vi "IR - Stop - addon.vi"(10 "IR Sensors":dbl[](array[numeric]), 11 "element":T1) -> (2 "appended array":dbl[](array[numeric]), 3 "0, 1":i16)   [LabVIEW 2019]
panel:
  out "Min":dbl
  out "Max":dbl
  out "logical AND":bool
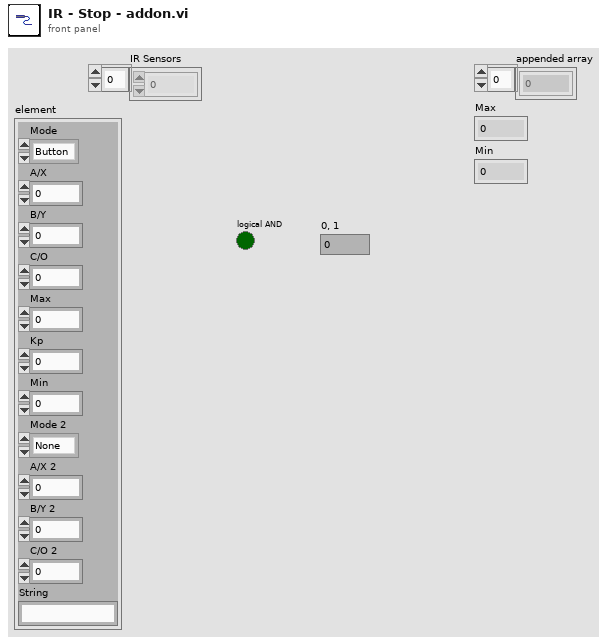
[diagram p1: front panel]
types:
  T1 = cluster{"Mode":enum16{"Button", "Encoder", "Delay", "IR Stop", "Line Stop"}, "A/X":dbl, "B/Y":dbl, "C/O":dbl, "Max":dbl, "Kp":dbl, "Min":dbl, "Mode 2":enum16{"None", "IR Stabilize", "Line Stabilize", "Encoder", "IR Stop", "Servo"}, "A/X 2":dbl, "B/Y 2":dbl, "C/O 2":dbl, "String":string}
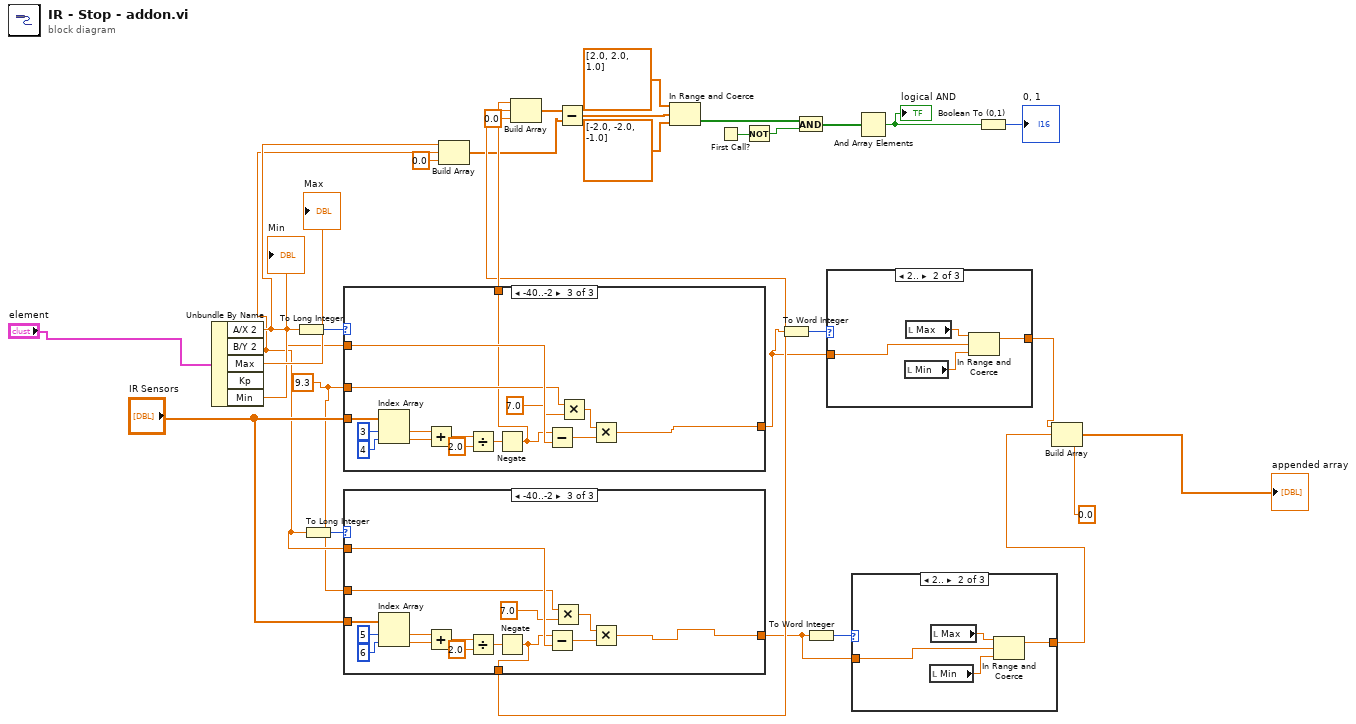
[diagram p0: block diagram]
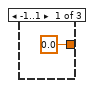
[diagram p2: hidden frame]
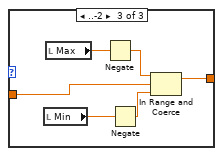
[diagram p3: hidden frame]
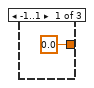
[diagram p4: hidden frame]
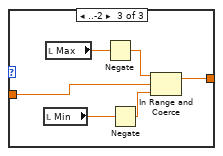
[diagram p5: hidden frame]
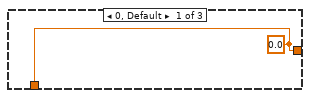
[diagram p6: hidden frame]
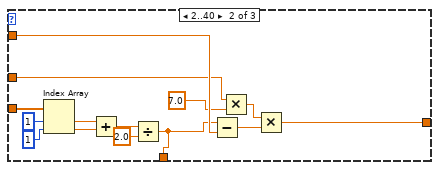
[diagram p7: hidden frame]
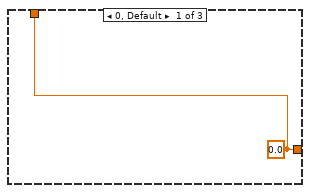
[diagram p8: hidden frame]
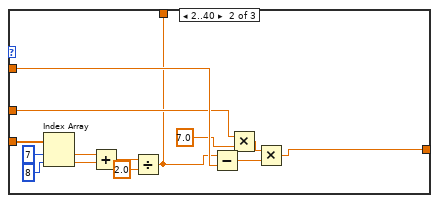
[diagram p9: hidden frame]
diagram:
  w2 = 9.3 ("Kp")
  n1 = Unbundle By Name("element") -> ("A/X 2"=w7:dbl, "B/Y 2"=w6:dbl, "Max"=→"Max":dbl, "Min"=→"Min":dbl)  [unwired: 1 out]
  n2 = To Long Integer(number=w7) -> (32bit integer=w32:i32)
  n3 = To Long Integer(number=w6) -> (32bit integer=w31:i32)
  n4 = case shown="-40..-2" w32 {
    tunnel: "IR Sensors" -> [_ w47 w62]
    tunnel: w7 -> [_ w40 w55]
    tunnel: w2 -> [_ w37 w51]
    tunnel: [w33 w34 w49] -> w9
    tunnel: [w33 w35 w48] -> w19
    frame 0, Default {
      w33 = 0.0 ("Max")
    }
    frame 2..40 {
      n5 = Index Array(array=w47, index #1=7 ("index"), index #2=8 ("index")) -> (element #1=w44:dbl, element #2=w43:dbl)
      n6 = Add(x=w44, y=w43) -> (x+y=w42:dbl)
      n7 = Divide(x=w42, y=2.0) -> (x/y=w35:dbl)
      n8 = Subtract(x=w35, y=w40) -> (x-y=w39:dbl)
      n9 = Multiply(x=w37, y=7.0) -> (x*y=w38:dbl)
      n10 = Multiply(x=w38, y=w39) -> (x*y=w34:dbl)
    }
    frame -40..-2 {
      n11 = Index Array(array=w62, index #1=3 ("index"), index #2=4 ("index")) -> (element #1=w59:dbl, element #2=w58:dbl)
      n12 = Add(x=w59, y=w58) -> (x+y=w57:dbl)
      n13 = Divide(x=w57, y=2.0) -> (x/y=w50:dbl)
      n14 = Negate(x=w50) -> (-x=w48:dbl)
      n15 = Subtract(x=w48, y=w55) -> (x-y=w54:dbl)
      n16 = Multiply(x=w51, y=7.0) -> (x*y=w52:dbl)
      n17 = Multiply(x=w52, y=w54) -> (x*y=w49:dbl)
    }
  }
  n18 = case shown="-40..-2" w31 {
    tunnel: "IR Sensors" -> [_ w77 w92]
    tunnel: w6 -> [_ w70 w85]
    tunnel: w2 -> [_ w66 w81]
    tunnel: [w63 w64 w79] -> w13
    tunnel: [w63 w65 w78] -> w18
    frame 0, Default {
      w63 = 0.0 ("Max")
    }
    frame 2..40 {
      n19 = Index Array(array=w77, index #1=1 ("index"), index #2=1 ("index")) -> (element #1=w74:dbl, element #2=w73:dbl)
      n20 = Add(x=w74, y=w73) -> (x+y=w72:dbl)
      n21 = Divide(x=w72, y=2.0) -> (x/y=w65:dbl)
      n22 = Subtract(x=w65, y=w70) -> (x-y=w69:dbl)
      n23 = Multiply(x=w66, y=7.0) -> (x*y=w67:dbl)
      n24 = Multiply(x=w67, y=w69) -> (x*y=w64:dbl)
    }
    frame -40..-2 {
      n25 = Index Array(array=w92, index #1=5 ("index"), index #2=6 ("index")) -> (element #1=w89:dbl, element #2=w88:dbl)
      n26 = Add(x=w89, y=w88) -> (x+y=w87:dbl)
      n27 = Divide(x=w87, y=2.0) -> (x/y=w80:dbl)
      n28 = Negate(x=w80) -> (-x=w78:dbl)
      n29 = Subtract(x=w78, y=w85) -> (x-y=w84:dbl)
      n30 = Multiply(x=w81, y=7.0) -> (x*y=w82:dbl)
      n31 = Multiply(x=w82, y=w84) -> (x*y=w79:dbl)
    }
  }
  n32 = Build Array(w7, w6, 0.0 ("element")) -> (w4:dbl[])
  n33 = Build Array(w19, w18, 0.0 ("element")) -> (w8:dbl[])
  n34 = Subtract(x=w8, y=w4) -> (x-y=w3:dbl[])
  n35 = In Range and Coerce(upper limit=dbl[] [2.0, 2.0, 1.0], x=w3, lower limit=dbl[] [-2.0, -2.0, -1.0]) -> (In Range?=w26:bool[])  [unwired: 1 out]
  n36 = First Call?() -> (First Call?: T/F=w25:bool)
  n37 = Not(x=w25) -> (.not. x?=w24:bool)
  n38 = To Word Integer(number=w9) -> (16bit integer=w11:i16)
  n39 = And(x=w26, y=w24) -> (x .and. y?=w23:bool[])
  n40 = To Word Integer(number=w13) -> (16bit integer=w14:i16)
  n41 = case shown="2.." w11 {
    tunnel: w9 -> [_ w95 w102]
    tunnel: [0.0 ("Max") w94 w101] -> w10
    frame -1..1 {
    }
    frame 2.. {
      n42 = local read "Min"() -> (w96:dbl)
      n43 = local read "Max"() -> (w97:dbl)
      n44 = In Range and Coerce(upper limit=w97, x=w95, lower limit=w96) -> (coerced(x)=w94:dbl)  [unwired: 1 out]
    }
    frame ..-2 {
      n45 = local read "Min"() -> (w100:dbl)
      n46 = local read "Max"() -> (w103:dbl)
      n47 = Negate(x=w103) -> (-x=w98:dbl)
      n48 = Negate(x=w100) -> (-x=w99:dbl)
      n49 = In Range and Coerce(upper limit=w98, x=w102, lower limit=w99) -> (coerced(x)=w101:dbl)  [unwired: 1 out]
    }
  }
  n50 = case shown="2.." w14 {
    tunnel: w13 -> [_ w106 w113]
    tunnel: [0.0 ("Max") w105 w112] -> w12
    frame -1..1 {
    }
    frame 2.. {
      n51 = local read "Min"() -> (w107:dbl)
      n52 = local read "Max"() -> (w108:dbl)
      n53 = In Range and Coerce(upper limit=w108, x=w106, lower limit=w107) -> (coerced(x)=w105:dbl)  [unwired: 1 out]
    }
    frame ..-2 {
      n54 = local read "Min"() -> (w111:dbl)
      n55 = local read "Max"() -> (w114:dbl)
      n56 = Negate(x=w114) -> (-x=w109:dbl)
      n57 = Negate(x=w111) -> (-x=w110:dbl)
      n58 = In Range and Coerce(upper limit=w109, x=w113, lower limit=w110) -> (coerced(x)=w112:dbl)  [unwired: 1 out]
    }
  }
  n59 = And Array Elements(Boolean array=w23) -> (logical AND=w22:bool)
  "logical AND" <- w22
  n60 = Boolean To (0,1)(Boolean=w22) -> (0, 1=→"0, 1":i16)
  n61 = Build Array(w10, w12, 0.0 ("element")) -> (→"appended array":dbl[])
